vi "load_configuration.vi"(2 "Cluster":T2, 3 "Handle":i32) -> (0 "output cluster":T3, 1 "output cluster":T2)   [LabVIEW 2010]
uses:
  <vilib>/Utility/xml.llb/Read From XML File(string).vi
panel:
  in  "XML input type":T1
  out "error out":errorcluster
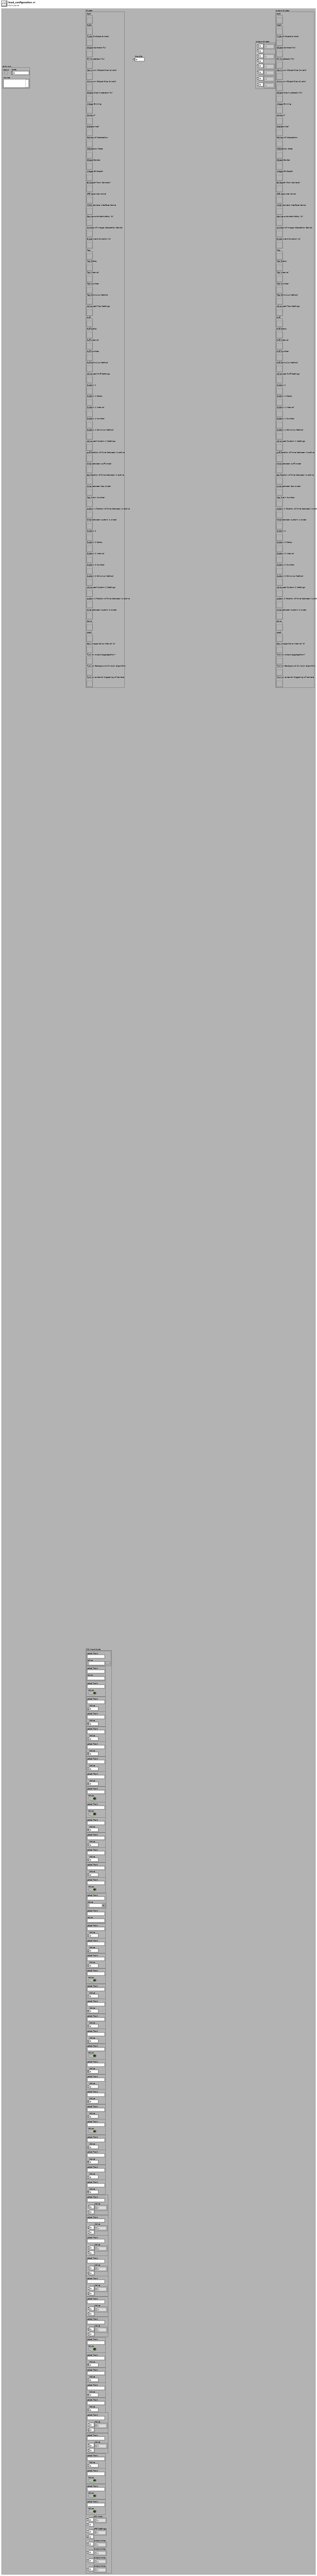
[diagram p1: front panel]
types:
  T1 = cluster{cluster{"Label.Text":string, "Value":path}, cluster{"Label.Text":string, "Value":string}, cluster{"Label.Text":string, "Value":bool}, cluster{"Label.Text":string, "Value":dbl}, cluster{"Label.Text":string, "Value":dbl}, cluster{"Label.Text":string, "Value":i32}, cluster{"Label.Text":string, "Value":i32}, cluster{"Label.Text":string, "Value":dbl}, cluster{"Label.Text":string, "Value":u16}, cluster{"Label.Text":string, "Value":bool}, cluster{"Label.Text":string, "Value":bool}, cluster{"Label.Text":string, "Value":i32}, cluster{"Label.Text":string, "Value":i32}, cluster{"Label.Text":string, "Value":i32}, cluster{"Label.Text":string, "Value":u32}, cluster{"Label.Text":string, "Value":bool}, cluster{"Label.Text":string, "Value":refnum<k15>}, cluster{"Label.Text":string, "Value":string}, cluster{"Label.Text":string, "Value":i32}, cluster{"Label.Text":string, "Value":i32}, cluster{"Label.Text":string, "Value":dbl}, cluster{"Label.Text":string, "Value":bool}, cluster{"Label.Text":string, "Value":dbl}, cluster{"Label.Text":string, "Value":dbl}, cluster{"Label.Text":string, "Value":i32}, cluster{"Label.Text":string, "Value":u16}, cluster{"Label.Text":string, "Value":bool}, cluster{"Label.Text":string, "Value":dbl}, cluster{"Label.Text":string, "Value":dbl}, cluster{"Label.Text":string, "Value":i32}, cluster{"Label.Text":string, "Value":u16}, cluster{"Label.Text":string, "Value":bool}, cluster{"Label.Text":string, "Value":dbl}, cluster{"Label.Text":string, "Value":dbl}, cluster{"Label.Text":string, "Value":i32}, cluster{"Label.Text":string, "Value":u16}, cluster{"Label.Text":string, "Value":sgl[][]}, cluster{"Label.Text":string, "Value":i32[][]}, cluster{"Label.Text":string, "Value":sgl[][]}, cluster{"Label.Text":string, "Value":i32[][]}, cluster{"Label.Text":string, "Value":i32[][]}, cluster{"Label.Text":string, "Value":sgl[][]}, cluster{"Label.Text":string, "Value":i32[][]}, cluster{"Label.Text":string, "Value":bool}, cluster{"Label.Text":string, "Value":dbl}, cluster{"Label.Text":string, "Value":dbl}, cluster{"Label.Text":string, "Value":i32}, cluster{"Label.Text":string, "Value":u16}, cluster{"Label.Text":string, "Value":sgl[][]}, cluster{"Label.Text":string, "Value":i32[][]}, cluster{"Label.Text":string, "Value":dbl}, cluster{"Label.Text":string, "Value":bool}, cluster{"Label.Text":string, "Value":bool}, cluster{"Label.Text":string, "Value":bool}, "ROI Array":dbl[][], "AFG Settings":dbl[][], "Output Array":dbl[], "Output Array":dbl[], "Output Array":dbl[], "Output Array":dbl[]}
  T2 = cluster{"Path":refnum<vi>, "Prefix":refnum<vi>, "Type of object to track":refnum<vi>, "Object Contrast (%)":refnum<vi>, "Fill Hysteresis (%)":refnum<vi>, "Maximum Object Size (pixels)":refnum<vi>, "Minimum Object Size (pixels)":refnum<vi>, "Object Size hysteresis (%)":refnum<vi>, "Image Binning":refnum<vi>, "Contour?":refnum<vi>, "Skeletonize?":refnum<vi>, "Frames of Adaptation":refnum<vi>, "Adaptation Rate":refnum<vi>, "Object Border":refnum<vi>, "Image Bit Depth":refnum<vi>, "Bit Depth from Camera?":refnum<vi>, "AFG resource name":refnum<vi>, "IMAQ Camera Interface Name":refnum<vi>, "Device auto-start delay (s)":refnum<vi>, "Number of Image Adaptation Bands":refnum<vi>, "Experiment Duration (s)":refnum<vi>, "Tap":refnum<vi>, "Tap Delay":refnum<vi>, "Tap Interval":refnum<vi>, "Tap Number":refnum<vi>, "Tap Stimulus Method":refnum<vi>, "Advanced Tap Settings":refnum<vi>, "Puff":refnum<vi>, "Puff Delay":refnum<vi>, "Puff Interval":refnum<vi>, "Puff Number":refnum<vi>, "Puff Stimulus Method":refnum<vi>, "Advanced Puff Settings":refnum<vi>, "Custom 1":refnum<vi>, "Custom 1 Delay":refnum<vi>, "Custom 1 Interval":refnum<vi>, "Custom 1 Number":refnum<vi>, "Custom 1 Stimulus Method":refnum<vi>, "Advanced Custom 1 Settings":refnum<vi>, "puff fraction of time between is active":refnum<vi>, "time between puff onset":refnum<vi>, "tap fraction of time between is active":refnum<vi>, "time between tap onset":refnum<vi>, "Tap Train Number":refnum<vi>, "custom 1 fraction of time between is active":refnum<vi>, "time between custom 1 onset":refnum<vi>, "Custom 2":refnum<vi>, "Custom 2 Delay":refnum<vi>, "Custom 2 Interval":refnum<vi>, "Custom 2 Number":refnum<vi>, "Custom 2 Stimulus Method":refnum<vi>, "Advanced Custom 2 Settings":refnum<vi>, "custom 2 fraction of time between is active":refnum<vi>, "time between custom 2 onset":refnum<vi>, "Save":refnum<vi>, "Load":refnum<vi>, "Raw Image Save Interval (s)":refnum<vi>, "Turn on output aggregation?":refnum<vi>, "Turn on Background division algorithm":refnum<vi>, "Turn on external triggering of camera":refnum<vi>}
  T3 = cluster{dbl[][], dbl[][], dbl[], dbl[], dbl[], dbl[]}
  T4 = cluster{"Label.Text":string, "Value":refnum<k15>}
  T5 = cluster{"ROI Array":dbl[][], "AFG Settings":dbl[][], "Output Array":dbl[], "Output Array":dbl[], "Output Array":dbl[], "Output Array":dbl[]}
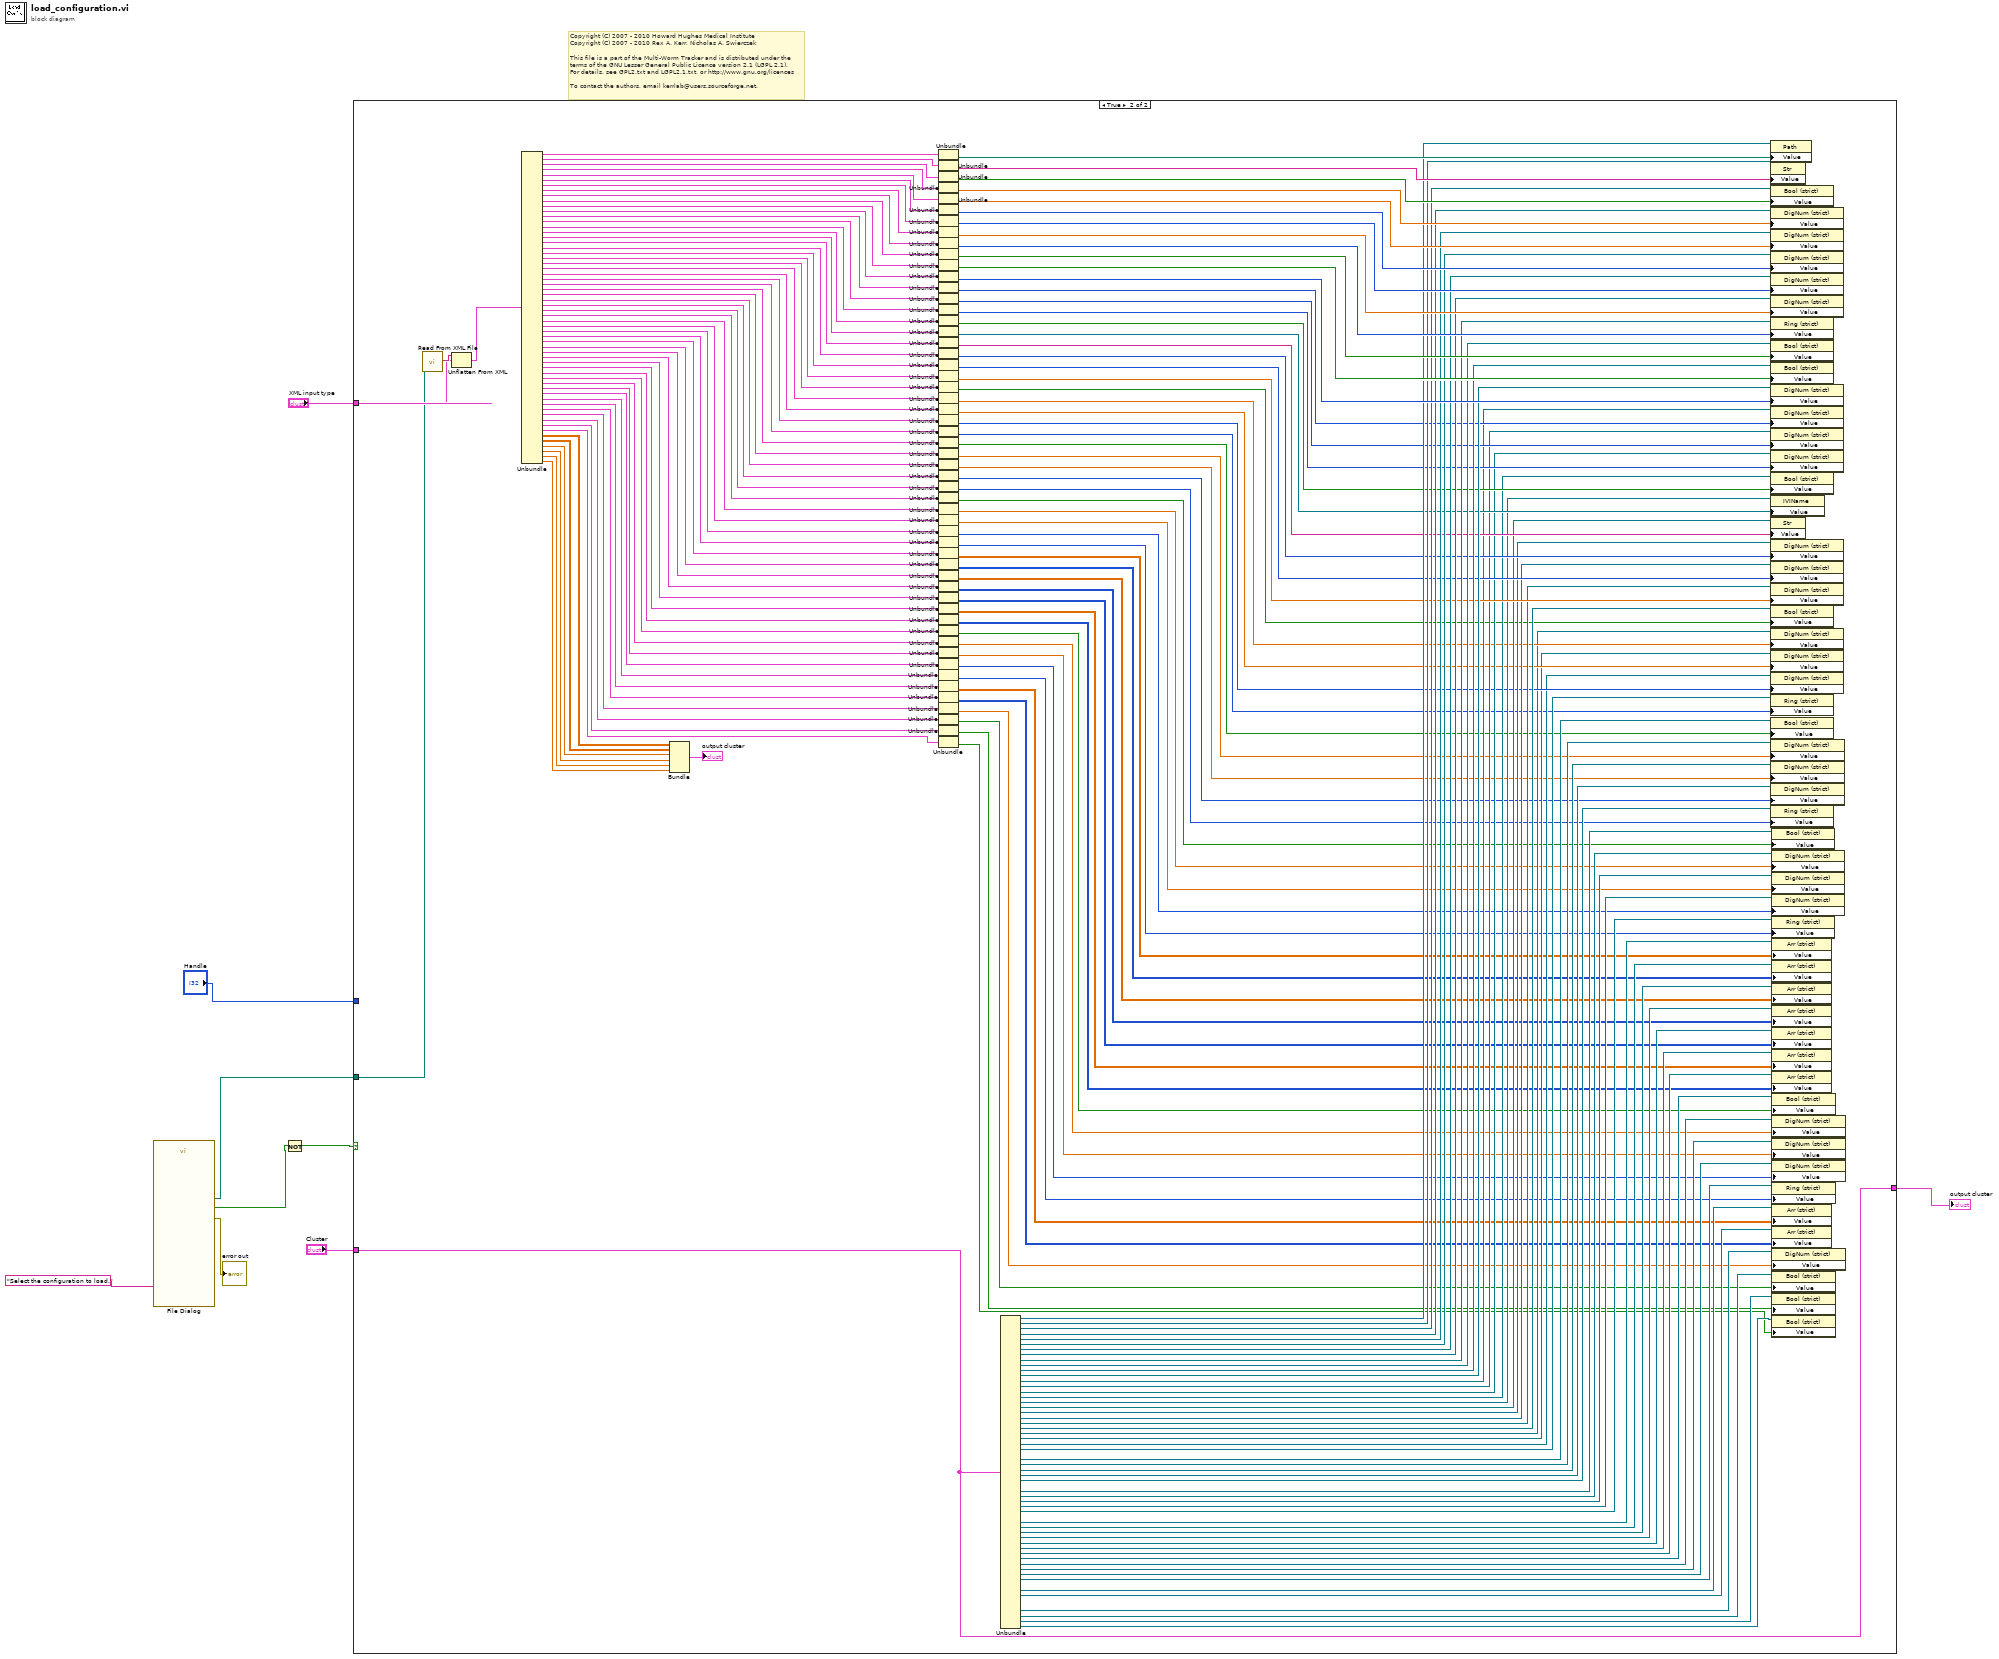
[diagram p0: block diagram]
diagram:
  # "Copyright (C) 2007 - 2010 Howard Hughes Medical Institute\nCopyright (C) 2007 - 2010 Rex A. Kerr, Nicholas A. Swierczek\n \nThis file is a part of the Multi-Worm Tracker and is distributed under the\nterms of the GNU Lesser General Public Licence version 2.1 (LGPL 2.1).\nFor details, see GPL2.txt and LGPL2.1.txt, or http://www.gnu.org/licences\n \nTo contact the authors, email kerrlab@users.sourceforge.net."
  n1 = call "File Dialog"("prompt"="Select the configuration to load.") -> ("selected path"=w3:path, "cancelled"=w7:bool, "error out"=→"error out":errorcluster)  [unwired: 11 in, 1 out]
  n2 = Not(x=w7) -> (.not. x?=w8:bool)
  n3 = case shown="True" w8 {
    tunnel: "Handle" -> [_ _]
    tunnel: [w10 w20] -> w4
    tunnel: "Cluster" -> [w10 w20]
    tunnel: w3 -> [_ w184]
    tunnel: "XML input type" -> [_ w182]
    frame False {
    }
    frame True {
      n4 = call-poly <vilib>:"Read From XML File.vi"("XML File Path"=w184) -> ("XML Elements"=w183:string)  [unwired: 8 in, 2 out]
      n5 = Unflatten From XML(xml string=w183, type=w182) -> (value=w92:T1)  [unwired: 1 in, 1 out]
      n6 = Unbundle(w92) -> (w181:cluster{"Label.Text":string, "Value":path}, w180:cluster{"Label.Text":string, "Value":string}, w179:cluster{"Label.Text":string, "Value":bool}, w178:cluster{"Label.Text":string, "Value":dbl}, w177:cluster{"Label.Text":string, "Value":dbl}, w176:cluster{"Label.Text":string, "Value":i32}, w175:cluster{"Label.Text":string, "Value":i32}, w174:cluster{"Label.Text":string, "Value":dbl}, w173:cluster{"Label.Text":string, "Value":u16}, w172:cluster{"Label.Text":string, "Value":bool}, w171:cluster{"Label.Text":string, "Value":bool}, w170:cluster{"Label.Text":string, "Value":i32}, w169:cluster{"Label.Text":string, "Value":i32}, w168:cluster{"Label.Text":string, "Value":i32}, w167:cluster{"Label.Text":string, "Value":u32}, w166:cluster{"Label.Text":string, "Value":bool}, w165:T4, w164:cluster{"Label.Text":string, "Value":string}, w163:cluster{"Label.Text":string, "Value":i32}, w162:cluster{"Label.Text":string, "Value":i32}, w161:cluster{"Label.Text":string, "Value":dbl}, w160:cluster{"Label.Text":string, "Value":bool}, w159:cluster{"Label.Text":string, "Value":dbl}, w158:cluster{"Label.Text":string, "Value":dbl}, w157:cluster{"Label.Text":string, "Value":i32}, w156:cluster{"Label.Text":string, "Value":u16}, w155:cluster{"Label.Text":string, "Value":bool}, w154:cluster{"Label.Text":string, "Value":dbl}, w153:cluster{"Label.Text":string, "Value":dbl}, w152:cluster{"Label.Text":string, "Value":i32}, w151:cluster{"Label.Text":string, "Value":u16}, w150:cluster{"Label.Text":string, "Value":bool}, w149:cluster{"Label.Text":string, "Value":dbl}, w148:cluster{"Label.Text":string, "Value":dbl}, w147:cluster{"Label.Text":string, "Value":i32}, w146:cluster{"Label.Text":string, "Value":u16}, w145:cluster{"Label.Text":string, "Value":sgl[][]}, w144:cluster{"Label.Text":string, "Value":i32[][]}, w143:cluster{"Label.Text":string, "Value":sgl[][]}, w142:cluster{"Label.Text":string, "Value":i32[][]}, w141:cluster{"Label.Text":string, "Value":i32[][]}, w140:cluster{"Label.Text":string, "Value":sgl[][]}, w139:cluster{"Label.Text":string, "Value":i32[][]}, w138:cluster{"Label.Text":string, "Value":bool}, w137:cluster{"Label.Text":string, "Value":dbl}, w136:cluster{"Label.Text":string, "Value":dbl}, w135:cluster{"Label.Text":string, "Value":i32}, w33:cluster{"Label.Text":string, "Value":u16}, w32:cluster{"Label.Text":string, "Value":sgl[][]}, w31:cluster{"Label.Text":string, "Value":i32[][]}, w30:cluster{"Label.Text":string, "Value":dbl}, w29:cluster{"Label.Text":string, "Value":bool}, w28:cluster{"Label.Text":string, "Value":bool}, w12:cluster{"Label.Text":string, "Value":bool}, "ROI Array"=w13:dbl[][], "AFG Settings"=w14:dbl[][], "Output Array"=w15:dbl[], "Output Array"=w16:dbl[], "Output Array"=w17:dbl[], "Output Array"=w18:dbl[])
      n7 = Bundle("ROI Array"=w13, "AFG Settings"=w14, "Output Array"=w15, "Output Array"=w16, "Output Array"=w17, "Output Array"=w18) -> (→"output cluster":T5)  [unwired: 1 in]
      n8 = Unbundle(w33) -> ("Value"=w27:u16)  [unwired: 1 out]
      n9 = Unbundle(w32) -> ("Value"=w26:sgl[][])  [unwired: 1 out]
      n10 = Unbundle(w31) -> ("Value"=w25:i32[][])  [unwired: 1 out]
      n11 = Unbundle(w30) -> ("Value"=w24:dbl)  [unwired: 1 out]
      n12 = Unbundle(w29) -> ("Value"=w23:bool)  [unwired: 1 out]
      n13 = Unbundle(w28) -> ("Value"=w22:bool)  [unwired: 1 out]
      n14 = Unbundle(w12) -> ("Value"=w11:bool)  [unwired: 1 out]
      n15 = Unbundle(w181) -> ("Value"=w134:path)  [unwired: 1 out]
      n16 = Unbundle(w180) -> ("Value"=w133:string)  [unwired: 1 out]
      n17 = Unbundle(w179) -> ("Value"=w132:bool)  [unwired: 1 out]
      n18 = Unbundle(w178) -> ("Value"=w131:dbl)  [unwired: 1 out]
      n19 = Unbundle(w177) -> ("Value"=w130:dbl)  [unwired: 1 out]
      n20 = Unbundle(w176) -> ("Value"=w129:i32)  [unwired: 1 out]
      n21 = Unbundle(w175) -> ("Value"=w128:i32)  [unwired: 1 out]
      n22 = Unbundle(w174) -> ("Value"=w127:dbl)  [unwired: 1 out]
      n23 = Unbundle(w173) -> ("Value"=w126:u16)  [unwired: 1 out]
      n24 = Unbundle(w172) -> ("Value"=w125:bool)  [unwired: 1 out]
      n25 = Unbundle(w171) -> ("Value"=w124:bool)  [unwired: 1 out]
      n26 = Unbundle(w170) -> ("Value"=w123:i32)  [unwired: 1 out]
      n27 = Unbundle(w169) -> ("Value"=w110:i32)  [unwired: 1 out]
      n28 = Unbundle(w168) -> ("Value"=w109:i32)  [unwired: 1 out]
      n29 = Unbundle(w167) -> ("Value"=w108:u32)  [unwired: 1 out]
      n30 = Unbundle(w166) -> ("Value"=w107:bool)  [unwired: 1 out]
      n31 = Unbundle(w165) -> ("Value"=w106:refnum<k15>)  [unwired: 1 out]
      n32 = Unbundle(w164) -> ("Value"=w105:string)  [unwired: 1 out]
      n33 = Unbundle(w163) -> ("Value"=w104:i32)  [unwired: 1 out]
      n34 = Unbundle(w162) -> ("Value"=w103:i32)  [unwired: 1 out]
      n35 = Unbundle(w161) -> ("Value"=w102:dbl)  [unwired: 1 out]
      n36 = Unbundle(w160) -> ("Value"=w90:bool)  [unwired: 1 out]
      n37 = Unbundle(w159) -> ("Value"=w89:dbl)  [unwired: 1 out]
      n38 = Unbundle(w158) -> ("Value"=w88:dbl)  [unwired: 1 out]
      n39 = Unbundle(w157) -> ("Value"=w87:i32)  [unwired: 1 out]
      n40 = Unbundle(w156) -> ("Value"=w82:u16)  [unwired: 1 out]
      n41 = Unbundle(w155) -> ("Value"=w54:bool)  [unwired: 1 out]
      n42 = Unbundle(w154) -> ("Value"=w53:dbl)  [unwired: 1 out]
      n43 = Unbundle(w153) -> ("Value"=w52:dbl)  [unwired: 1 out]
      n44 = Unbundle(w152) -> ("Value"=w51:i32)  [unwired: 1 out]
      n45 = Unbundle(w151) -> ("Value"=w50:u16)  [unwired: 1 out]
      n46 = Unbundle(w150) -> ("Value"=w49:bool)  [unwired: 1 out]
      n47 = Unbundle(w149) -> ("Value"=w48:dbl)  [unwired: 1 out]
      n48 = Unbundle(w148) -> ("Value"=w47:dbl)  [unwired: 1 out]
      n49 = Unbundle(w147) -> ("Value"=w46:i32)  [unwired: 1 out]
      n50 = Unbundle(w146) -> ("Value"=w45:u16)  [unwired: 1 out]
      n51 = Unbundle(w145) -> ("Value"=w44:sgl[][])  [unwired: 1 out]
      n52 = Unbundle(w144) -> ("Value"=w43:i32[][])  [unwired: 1 out]
      n53 = Unbundle(w143) -> ("Value"=w42:sgl[][])  [unwired: 1 out]
      n54 = Unbundle(w142) -> ("Value"=w41:i32[][])  [unwired: 1 out]
      n55 = Unbundle(w141) -> ("Value"=w40:i32[][])  [unwired: 1 out]
      n56 = Unbundle(w140) -> ("Value"=w39:sgl[][])  [unwired: 1 out]
      n57 = Unbundle(w139) -> ("Value"=w38:i32[][])  [unwired: 1 out]
      n58 = Unbundle(w138) -> ("Value"=w37:bool)  [unwired: 1 out]
      n59 = Unbundle(w137) -> ("Value"=w36:dbl)  [unwired: 1 out]
      n60 = Unbundle(w136) -> ("Value"=w35:dbl)  [unwired: 1 out]
      n61 = Unbundle(w135) -> ("Value"=w34:i32)  [unwired: 1 out]
      n62 = Unbundle(w20) -> ("Path"=w122:refnum<vi>, "Prefix"=w121:refnum<vi>, "Type of object to track"=w120:refnum<vi>, "Object Contrast (%)"=w119:refnum<vi>, "Fill Hysteresis (%)"=w118:refnum<vi>, "Maximum Object Size (pixels)"=w117:refnum<vi>, "Minimum Object Size (pixels)"=w116:refnum<vi>, "Object Size hysteresis (%)"=w115:refnum<vi>, "Image Binning"=w114:refnum<vi>, "Contour?"=w113:refnum<vi>, "Skeletonize?"=w112:refnum<vi>, "Frames of Adaptation"=w111:refnum<vi>, "Adaptation Rate"=w101:refnum<vi>, "Object Border"=w100:refnum<vi>, "Image Bit Depth"=w99:refnum<vi>, "Bit Depth from Camera?"=w98:refnum<vi>, "AFG resource name"=w97:refnum<vi>, "IMAQ Camera Interface Name"=w96:refnum<vi>, "Device auto-start delay (s)"=w95:refnum<vi>, "Number of Image Adaptation Bands"=w94:refnum<vi>, "Experiment Duration (s)"=w93:refnum<vi>, "Tap"=w91:refnum<vi>, "Tap Delay"=w86:refnum<vi>, "Tap Interval"=w85:refnum<vi>, "Tap Number"=w84:refnum<vi>, "Tap Stimulus Method"=w83:refnum<vi>, "Puff"=w81:refnum<vi>, "Puff Delay"=w80:refnum<vi>, "Puff Interval"=w79:refnum<vi>, "Puff Number"=w78:refnum<vi>, "Puff Stimulus Method"=w77:refnum<vi>, "Custom 1"=w76:refnum<vi>, "Custom 1 Delay"=w75:refnum<vi>, "Custom 1 Interval"=w74:refnum<vi>, "Custom 1 Number"=w73:refnum<vi>, "Custom 1 Stimulus Method"=w72:refnum<vi>, "puff fraction of time between is active"=w71:refnum<vi>, "time between puff onset"=w70:refnum<vi>, "tap fraction of time between is active"=w69:refnum<vi>, "time between tap onset"=w68:refnum<vi>, "Tap Train Number"=w67:refnum<vi>, "custom 1 fraction of time between is active"=w66:refnum<vi>, "time between custom 1 onset"=w65:refnum<vi>, "Custom 2"=w64:refnum<vi>, "Custom 2 Delay"=w63:refnum<vi>, "Custom 2 Interval"=w62:refnum<vi>, "Custom 2 Number"=w61:refnum<vi>, "Custom 2 Stimulus Method"=w60:refnum<vi>, "custom 2 fraction of time between is active"=w59:refnum<vi>, "time between custom 2 onset"=w58:refnum<vi>, "Raw Image Save Interval (s)"=w57:refnum<vi>, "Turn on output aggregation?"=w56:refnum<vi>, "Turn on Background division algorithm"=w55:refnum<vi>, "Turn on external triggering of camera"=w19:refnum<vi>)  [unwired: 6 out]
      n63 = property class="Path"(reference=w122, "Value"=w134) -> ()  [unwired: 1 in, 2 out]
      n64 = property class="Str"(reference=w121, "Value"=w133) -> ()  [unwired: 1 in, 2 out]
      n65 = property class="Bool (strict)"(reference=w120, "Value"=w132) -> ()  [unwired: 1 in, 2 out]
      n66 = property class="DigNum (strict)"(reference=w119, "Value"=w131) -> ()  [unwired: 1 in, 2 out]
      n67 = property class="DigNum (strict)"(reference=w118, "Value"=w130) -> ()  [unwired: 1 in, 2 out]
      n68 = property class="DigNum (strict)"(reference=w117, "Value"=w129) -> ()  [unwired: 1 in, 2 out]
      n69 = property class="DigNum (strict)"(reference=w116, "Value"=w128) -> ()  [unwired: 1 in, 2 out]
      n70 = property class="DigNum (strict)"(reference=w115, "Value"=w127) -> ()  [unwired: 1 in, 2 out]
      n71 = property class="Ring (strict)"(reference=w114, "Value"=w126) -> ()  [unwired: 1 in, 2 out]
      n72 = property class="Bool (strict)"(reference=w113, "Value"=w125) -> ()  [unwired: 1 in, 2 out]
      n73 = property class="Bool (strict)"(reference=w112, "Value"=w124) -> ()  [unwired: 1 in, 2 out]
      n74 = property class="DigNum (strict)"(reference=w111, "Value"=w123) -> ()  [unwired: 1 in, 2 out]
      n75 = property class="DigNum (strict)"(reference=w101, "Value"=w110) -> ()  [unwired: 1 in, 2 out]
      n76 = property class="DigNum (strict)"(reference=w100, "Value"=w109) -> ()  [unwired: 1 in, 2 out]
      n77 = property class="DigNum (strict)"(reference=w99, "Value"=w108) -> ()  [unwired: 1 in, 2 out]
      n78 = property class="Bool (strict)"(reference=w98, "Value"=w107) -> ()  [unwired: 1 in, 2 out]
      n79 = property class="IVIName"(reference=w97, "Value"=w106) -> ()  [unwired: 1 in, 2 out]
      n80 = property class="Str"(reference=w96, "Value"=w105) -> ()  [unwired: 1 in, 2 out]
      n81 = property class="DigNum (strict)"(reference=w95, "Value"=w104) -> ()  [unwired: 1 in, 2 out]
      n82 = property class="DigNum (strict)"(reference=w94, "Value"=w103) -> ()  [unwired: 1 in, 2 out]
      n83 = property class="DigNum (strict)"(reference=w93, "Value"=w102) -> ()  [unwired: 1 in, 2 out]
      n84 = property class="Bool (strict)"(reference=w91, "Value"=w90) -> ()  [unwired: 1 in, 2 out]
      n85 = property class="DigNum (strict)"(reference=w86, "Value"=w89) -> ()  [unwired: 1 in, 2 out]
      n86 = property class="DigNum (strict)"(reference=w85, "Value"=w88) -> ()  [unwired: 1 in, 2 out]
      n87 = property class="DigNum (strict)"(reference=w84, "Value"=w87) -> ()  [unwired: 1 in, 2 out]
      n88 = property class="Ring (strict)"(reference=w83, "Value"=w82) -> ()  [unwired: 1 in, 2 out]
      n89 = property class="Bool (strict)"(reference=w81, "Value"=w54) -> ()  [unwired: 1 in, 2 out]
      n90 = property class="DigNum (strict)"(reference=w80, "Value"=w53) -> ()  [unwired: 1 in, 2 out]
      n91 = property class="DigNum (strict)"(reference=w79, "Value"=w52) -> ()  [unwired: 1 in, 2 out]
      n92 = property class="DigNum (strict)"(reference=w78, "Value"=w51) -> ()  [unwired: 1 in, 2 out]
      n93 = property class="Ring (strict)"(reference=w77, "Value"=w50) -> ()  [unwired: 1 in, 2 out]
      n94 = property class="Bool (strict)"(reference=w76, "Value"=w49) -> ()  [unwired: 1 in, 2 out]
      n95 = property class="DigNum (strict)"(reference=w75, "Value"=w48) -> ()  [unwired: 1 in, 2 out]
      n96 = property class="DigNum (strict)"(reference=w74, "Value"=w47) -> ()  [unwired: 1 in, 2 out]
      n97 = property class="DigNum (strict)"(reference=w73, "Value"=w46) -> ()  [unwired: 1 in, 2 out]
      n98 = property class="Ring (strict)"(reference=w72, "Value"=w45) -> ()  [unwired: 1 in, 2 out]
      n99 = property class="Arr (strict)"(reference=w71, "Value"=w44) -> ()  [unwired: 1 in, 2 out]
      n100 = property class="Arr (strict)"(reference=w70, "Value"=w43) -> ()  [unwired: 1 in, 2 out]
      n101 = property class="Arr (strict)"(reference=w69, "Value"=w42) -> ()  [unwired: 1 in, 2 out]
      n102 = property class="Arr (strict)"(reference=w68, "Value"=w41) -> ()  [unwired: 1 in, 2 out]
      n103 = property class="Arr (strict)"(reference=w67, "Value"=w40) -> ()  [unwired: 1 in, 2 out]
      n104 = property class="Arr (strict)"(reference=w66, "Value"=w39) -> ()  [unwired: 1 in, 2 out]
      n105 = property class="Arr (strict)"(reference=w65, "Value"=w38) -> ()  [unwired: 1 in, 2 out]
      n106 = property class="Bool (strict)"(reference=w64, "Value"=w37) -> ()  [unwired: 1 in, 2 out]
      n107 = property class="DigNum (strict)"(reference=w63, "Value"=w36) -> ()  [unwired: 1 in, 2 out]
      n108 = property class="DigNum (strict)"(reference=w62, "Value"=w35) -> ()  [unwired: 1 in, 2 out]
      n109 = property class="DigNum (strict)"(reference=w61, "Value"=w34) -> ()  [unwired: 1 in, 2 out]
      n110 = property class="Ring (strict)"(reference=w60, "Value"=w27) -> ()  [unwired: 1 in, 2 out]
      n111 = property class="Arr (strict)"(reference=w59, "Value"=w26) -> ()  [unwired: 1 in, 2 out]
      n112 = property class="Arr (strict)"(reference=w58, "Value"=w25) -> ()  [unwired: 1 in, 2 out]
      n113 = property class="DigNum (strict)"(reference=w57, "Value"=w24) -> ()  [unwired: 1 in, 2 out]
      n114 = property class="Bool (strict)"(reference=w56, "Value"=w23) -> ()  [unwired: 1 in, 2 out]
      n115 = property class="Bool (strict)"(reference=w55, "Value"=w22) -> ()  [unwired: 1 in, 2 out]
      n116 = property class="Bool (strict)"(reference=w19, "Value"=w11) -> ()  [unwired: 1 in, 2 out]
    }
  }
  "output cluster" <- w4
